vi "abort_red_tweezers.vi"   [LabVIEW 2010]
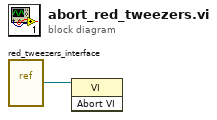
[diagram p0: block diagram]
diagram:
  n1 = vi-ref "red_tweezers_interface.vi"() -> (w1:refnum<vi>)
  n2 = invoke class="VI" method="Abort VI"(reference=w1) -> ()  [unwired: 2 in, 3 out]
